vi "Catch Nested Value Update.vi"(8 "error in (no error)":errorcluster, 10 "Nested Value Update Msg":refnum<class "Nested Value Update Msg.lvclass">, 11 "Process Builder ViewManager In":refnum<class "Navigation ViewManager.lvclass">) -> (0 "error out":errorcluster, 3 "Process Builder ViewManager Out":refnum<class "Navigation ViewManager.lvclass">)   [LabVIEW 2019, in "Navigation ViewManager.lvclass"]
doc: "<License>\nCopyright © 2017 Composed Systems, LLC | All rights reserved\nwww.composed.io\n\nAuthor: Ethan Stern <ethan.stern@composed.io>\n\nThis software is provided \"AS IS\" WITHOUT WARRANTIES, either express or implied, AND IS FOR EDUCATIONAL PURPOSES ONLY.\n</License>"
uses:
  <vilib>/gpm_packages/@cs/Car-wash/Source/Process Builder ViewManager/Navigation ViewManager.lvclass
  C:/Program Files/National Instruments/LabVIEW 2019/vi.lib/gpm_packages/@cs/mva-viewable/Source/IViewManager/IViewManager/IViewManager.lvclass
  <vilib>/gpm_packages/@cs/mva-viewable/Source/IViewable/IViewable Messages/Catch Nested Value Change Msg/Nested Value Update Msg.lvclass
  <vilib>/gpm_packages/@cs/mva-viewable/Source/IViewable/IViewable Messages/Catch Nested Value Change Msg/Nested Value Update Msg.lvclass/Nested Value Update Msg.ctl
  <vilib>/gpm_packages/@cs/mva-viewable/Source/IViewManager/IViewManager/IViewManager.lvclass/IViewManager.ctl
  <vilib>/gpm_packages/@cs/Car-wash/Source/Process Builder ViewManager/Navigation ViewManager.lvclass/Navigation ViewManager.ctl
  <vilib>/gpm_packages/@cs/mva-viewable/Source/IViewable/IViewable Messages/Insert Front Panel Msg/Insert Front Panel Msg.lvclass/Insert Front Panel Msg.ctl
  <vilib>/ActorFramework/Message Enqueuer/Message Enqueuer.lvclass/Message Enqueuer.ctl
  <vilib>/ActorFramework/Message Enqueuer/Enqueue.vi
  <vilib>/gpm_packages/@cs/mva-viewable/Source/IViewable/IViewable Messages/Insert Front Panel Msg/Insert Front Panel Msg.lvclass
  C:/Program Files/National Instruments/LabVIEW 2019/vi.lib/ActorFramework/Message/Message.lvclass
  <vilib>/ActorFramework/Message Priority Queue/Priority Enqueue.vi
  <vilib>/gpm_packages/@cs/mva-viewable/Source/IViewManager/IViewManager/IViewManager.lvclass
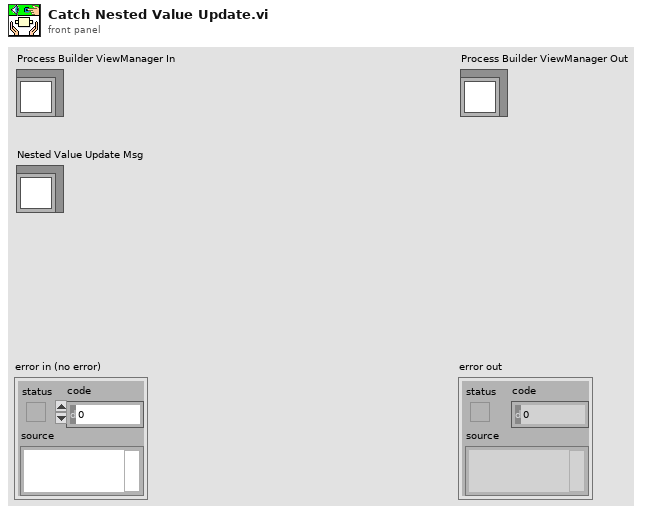
[diagram p1: front panel]
types:
  T1 = typedef "IViewable.lvlib/ProtectedSubpanel.lvclass/Protected Subpanel Reference.ctl" = refnum<data-value>
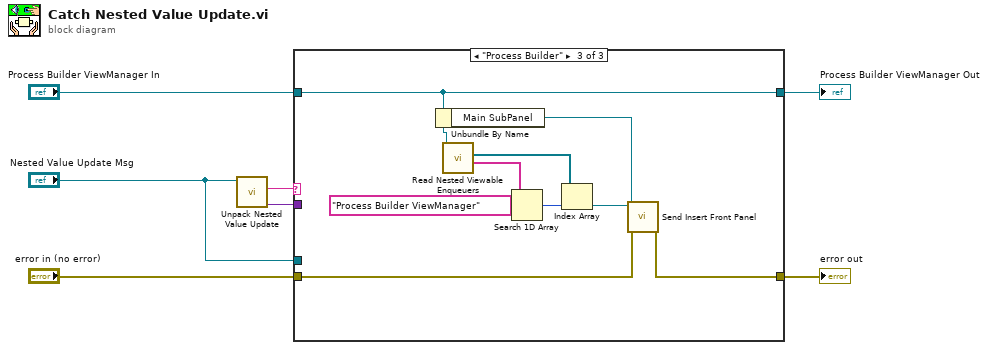
[diagram p0: block diagram]
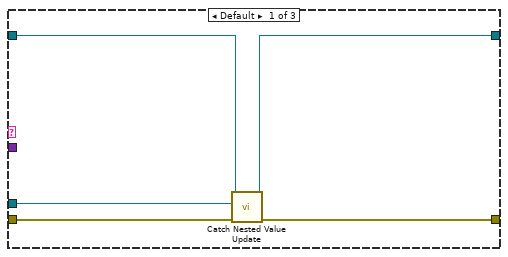
[diagram p2: hidden frame]
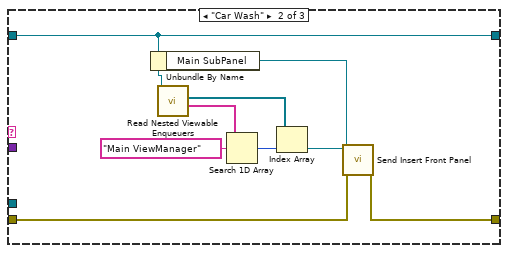
[diagram p3: hidden frame]
diagram:
  n1 = call <vilib>:"Unpack Nested Value Update.vi"("Nested Value Update Msg"="Nested Value Update Msg") -> ("Value"=w1:variant, "Datum Name"=w2:string)  [unwired: 8 in, 1 out]
  n2 = case shown="\"Process Builder\"" w2 {
    tunnel: [w12 w13 w22] -> w7
    tunnel: [w11 w17 w26] -> w6
    tunnel: "error in (no error)" -> [w10 w14 w23]
    tunnel: "Process Builder ViewManager In" -> [w9 w17 w26]
    tunnel: "Nested Value Update Msg" -> [w8 _ _]
    tunnel: w1 -> [_ _ _]
    frame Default {
      n3 = call-parent "Catch Nested Value Update.vi"("error in (no error)"=w10, "Nested Value Update Msg"=w8, "IViewable In"=w9) -> ("error out"=w12:errorcluster, "IViewable Out"=w11:refnum<class "Navigation ViewManager.lvclass">)  [unwired: 7 in]
    }
    frame "Car Wash" {
      n4 = Unbundle By Name(w17) -> ("Main SubPanel"=w16:T1)
      n5 = call <vilib>:"Read Nested Viewable Enqueuers.vi"("IViewManager in"=w17) -> ("Viewable Names"=w21:string[], "Nested Viewable Enqueuers"=w19:refnum<class "Message Enqueuer.lvclass">[])  [unwired: 9 in]
      n6 = Search 1D Array(1D array=w21, element="Main ViewManager") -> (index of element=w18:i32)  [unwired: 1 in]
      n7 = Index Array(array=w19, index=w18) -> (element=w15:refnum<class "Message Enqueuer.lvclass">)
      n8 = call <vilib>:"Send Insert Front Panel.vi"("error in (no error)"=w14, "Protected Subpanel"=w16, "Message Enqueuer"=w15) -> ("error out"=w13:errorcluster)  [unwired: 7 in, 1 out]
    }
    frame "Process Builder" {
      n9 = Unbundle By Name(w26) -> ("Main SubPanel"=w25:T1)
      n10 = call <vilib>:"Read Nested Viewable Enqueuers.vi"("IViewManager in"=w26) -> ("Viewable Names"=w30:string[], "Nested Viewable Enqueuers"=w28:refnum<class "Message Enqueuer.lvclass">[])  [unwired: 9 in]
      n11 = Search 1D Array(1D array=w30, element="Process Builder ViewManager") -> (index of element=w27:i32)  [unwired: 1 in]
      n12 = Index Array(array=w28, index=w27) -> (element=w24:refnum<class "Message Enqueuer.lvclass">)
      n13 = call <vilib>:"Send Insert Front Panel.vi"("error in (no error)"=w23, "Protected Subpanel"=w25, "Message Enqueuer"=w24) -> ("error out"=w22:errorcluster)  [unwired: 7 in, 1 out]
    }
  }
  "error out" <- w7
  "Process Builder ViewManager Out" <- w6
